vi "Main_Run.vi"() -> ()   [LabVIEW 2019, in "Motor_Lib.lvlib"]
uses:
  Motor_Lib.lvlib
  MotorType.ctl
  <vilib>/Platform/TimedLoop/XDataNode/timing_clust.ctl
  <vilib>/Platform/TimedLoop/XDataNode/nitl_modes.ctl
  <vilib>/Platform/TimedLoop/XDataNode/wakeup.ctl
  PORT_ID.ctl
  <vilib>/myRIO/Common/Instrument Driver Framework/myRIO v1.0/UART/vis/myRIO v1.0 Close UART.vi
  <vilib>/myRIO/Common/Instrument Driver Framework/Utilities/vis/FPGA Ref Manager.vi
  <vilib>/myRIO/Common/Instrument Driver Framework/myRIO v1.0/myRIO v1.0 Reset FPGA.vi
  <vilib>/myRIO/Common/Instrument Driver Framework/myRIO v1.0/IRQ/vis/myRIO v1.0 IRQ Info FGV.vi
  <vilib>/myRIO/Common/Instrument Driver Framework/myRIO v1.0/IRQ/vis/myRIO v1.0 Timer IRQ Info FGV.vi
  <vilib>/myRIO/Common/Instrument Driver Framework/myRIO v1.0/IRQ/vis/myRIO v1.0 ISR Agent.vi
  <vilib>/myRIO/Instrument Drivers/Utilities/vis/Reset Index.vi
  <vilib>/myRIO/Common/Instrument Driver Framework/myRIO v1.0/Resource Manager/vis/myRIO v1.0 Block Write Resource Manager.vi
  <vilib>/platform/TimedLoop/XDataNode/XDataNode.xnode
  <vilib>/Platform/TimedLoop/XDataNode/XDNodeRunTimeDep.lvlib
  <vilib>/myRIO/Instrument Drivers/Utilities/Utilities.lvlib
panel:
  in  "MotorA":T1=1 items=["BLDC", "BDC"]
  in  "TargetRPM(Motor A)":dbl format="%.2f"
  in  "ResetA":bool
  in  "MotorB":T1 items=["BLDC", "BDC"]
  in  "ResetB":bool
  in  "TargetRPM(Motor B)":dbl format="%.2f"
  out "RPM/T Chart(Motor B)":T2(graph)
  out "RPM/T Chart(Motor A)":cluster{"upper limit":dbl, "RPM":dbl}(graph)
  in  "stop":bool
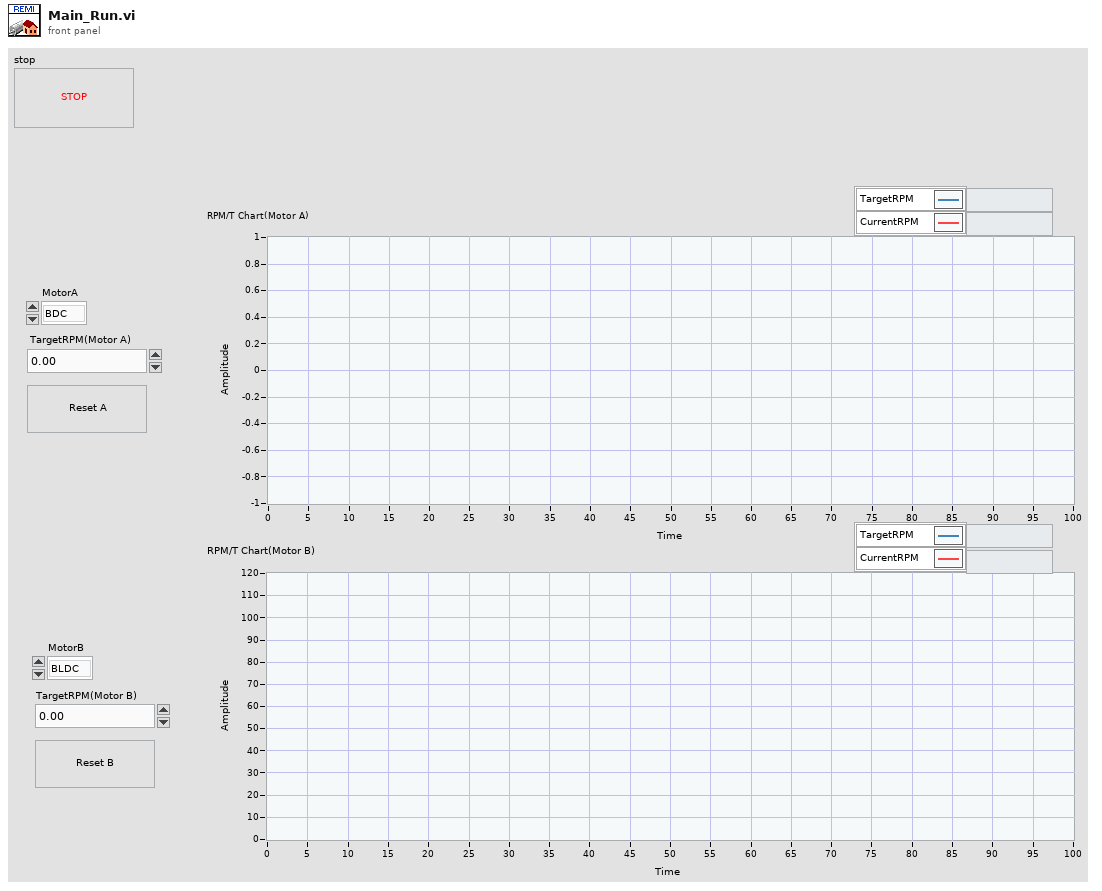
[diagram p1: front panel]
types:
  T1 = typedef "Motor_Lib.lvlib/MotorType.ctl" = u16
  T2 = cluster{"TargetRPM(Motor B)":dbl, "Rotations":dbl}
  T3 = typedef "Motor_Lib.lvlib/PORT_ID.ctl" = enum16{"PORT_A", "PORT_B"}
  T4 = typedef "XDNodeRunTimeDep.lvlib/timing_clust.ctl" = cluster{"Expected End [f-1]":u64, "Actual End [f-1]":u64, "Finished Late? [f-1]":bool, "Expected End [i-1]":u64, "Actual End [i-1]":u64, "Finished Late? [i-1]":bool, "Expected Start [i]":u64, "Actual Start [i]":u64, "Expected Start [f]":u64, "Actual Start [f]":u64, "Source Name":string, "Structure Name":string, "Period":i64, "Deadline":i64, "Offset":i64, "Start":i64, "Priority":i32, "Timeout":i32, "Mode":T5, "Wakeup Reason":T6, "Error":errorcluster, "Source Type":string, "Secondary Source Type":string, "Global End Time":u64, "Global Start Time":u64, "Frame Duration":u64, "Iteration Duration":u64, "Assigned CPU":i32, "I/O Scan Engine Mode":u32}
  T5 = typedef "XDNodeRunTimeDep.lvlib/nitl_modes.ctl" = enum32{"No Change", "Process missed periods, maintain original phase", "Discard missed periods, maintain original phase", "Process missed periods, ignore original phase", "Discard missed periods, ignore original phase"}
  T6 = typedef "XDNodeRunTimeDep.lvlib/wakeup.ctl" = enum32{"Normal", "Aborted", "Asynchronous wakeup", "Timing source error", "Timed loop error", "Timeout"}
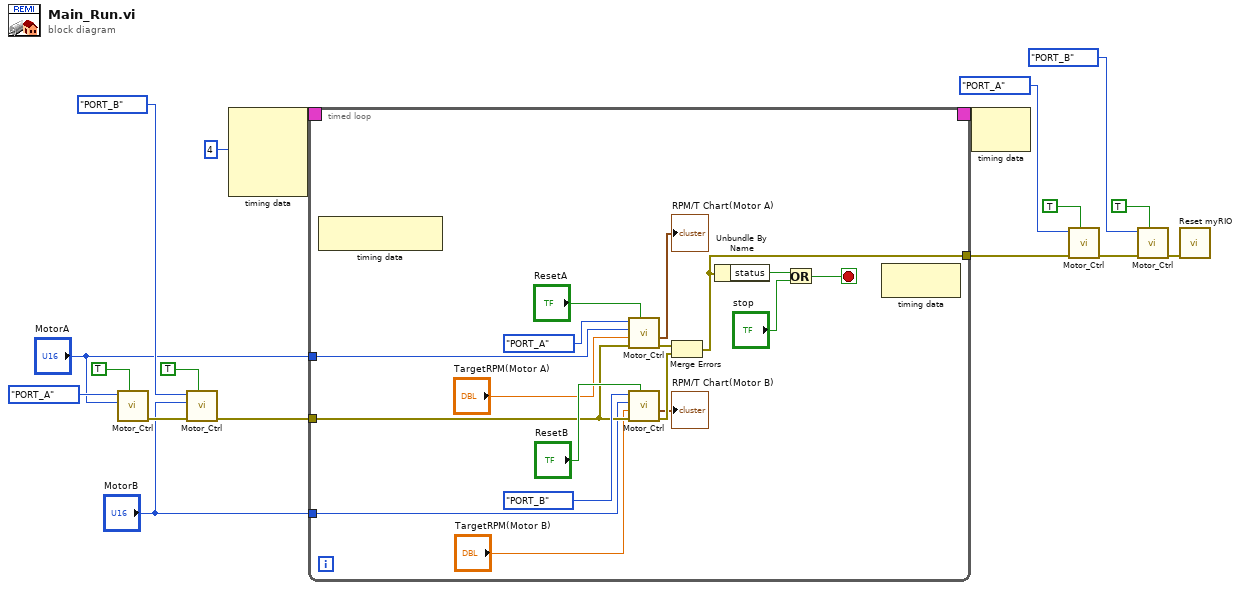
[diagram p0: block diagram]
diagram:
  n1 = call "Motor_Ctrl.vi"("Reset"=TRUE, "B/BL Motor"="MotorA", "Port"=PORT_ID."PORT_A") -> ("error out"=w4:errorcluster)  [unwired: 5 in, 3 out]
  n2 = call "Motor_Ctrl.vi"("Reset"=TRUE, "error in (no error)"=w4, "B/BL Motor"="MotorB", "Port"=PORT_ID."PORT_B") -> ("error out"=w3:errorcluster)  [unwired: 4 in, 3 out]
  n3 = node-c288(i64 4 ("Period")) -> (w18:T4)  [unwired: 3 in]
  n4 = timed-loop {
    timing: w18 -> [_]
    timing-out: [_] -> w17
    tunnel: [w30] -> w10
    tunnel: w3 -> [w24]
    tunnel: "MotorB" -> [w20]
    tunnel: "MotorA" -> [w19]
    stop <- w27 stop-if-true
    n5 = node-c288() -> ()  [unwired: 1 in, 1 out]
    n6 = call "Motor_Ctrl.vi"("Reset"="ResetA", "error in (no error)"=w24, "TargetRPM(+/-120)"="TargetRPM(Motor A)", "B/BL Motor"=w19, "Port"=PORT_ID."PORT_A" ("PORT")) -> ("error out"=w32:errorcluster, "RPM/T Chart"=→"RPM/T Chart(Motor A)":cluster{"upper limit":dbl, "RPM":dbl})  [unwired: 3 in, 2 out]
    n7 = call "Motor_Ctrl.vi"("Reset"="ResetB", "error in (no error)"=w24, "TargetRPM(+/-120)"="TargetRPM(Motor B)", "B/BL Motor"=w20, "Port"=PORT_ID."PORT_B" ("PORT")) -> ("error out"=w31:errorcluster, "RPM/T Chart"=→"RPM/T Chart(Motor B)":cluster{"upper limit":dbl, "RPM":dbl})  [unwired: 3 in, 2 out]
    n8 = Merge Errors(w32, w31) -> (w30:errorcluster)
    n9 = Unbundle By Name(w30) -> ("status"=w28:bool)
    n10 = Or(x=w28, y="stop") -> (x .or. y?=w27:bool)
    n11 = node-c288() -> ()  [unwired: 1 in, 1 out]
  }
  n12 = node-c288(w17) -> ()  [unwired: 1 out]
  n13 = call "Motor_Ctrl.vi"("Reset"=TRUE, "error in (no error)"=w10, "Port"=PORT_ID."PORT_A") -> ("error out"=w11:errorcluster)  [unwired: 5 in, 3 out]
  n14 = call "Motor_Ctrl.vi"("Reset"=TRUE, "error in (no error)"=w11, "Port"=PORT_ID."PORT_B") -> ("error out"=w9:errorcluster)  [unwired: 5 in, 3 out]
  n15 = call <vilib>:"Reset myRIO.vi"("error in (no error)"=w9) -> ()  [unwired: 10 in, 1 out]
